vi "Device Unload.vi"(8 "error in (no error)":errorcluster, 9 "IED Name":string, 11 "SCADA in":refnum<class "SCADA.lvclass">) -> (0 "error out":errorcluster, 3 "SCADA out":refnum<class "SCADA.lvclass">)   [LabVIEW 2015, in "SCADA Core.lvlib" / "SCADA.lvclass"]
uses:
  SCADA.lvclass
  Controls/Queue Selector.ctl
  <vilib>/ActorFramework/Actor/Actor.lvclass/Actor.ctl
  SCADA.lvclass/SCADA.ctl
  <vilib>/ActorFramework/Message Enqueuer/Message Enqueuer.lvclass/Message Enqueuer.ctl
  SCADA Abstract Messages/Device Action Status Msg/Device Action Status.ctl
  <vilib>/Utility/error.llb/DialogType.ctl
  <vilib>/ActorFramework/Message Enqueuer/Enqueue.vi
  <vilib>/ActorFramework/Message Priority Queue/Priority Enqueue.vi
  <vilib>/ActorFramework/Stop Msg/Stop Msg.lvclass
  <vilib>/ActorFramework/Actor/Actor.lvclass
  SCADA Abstract Messages/Device Action Status Msg/Device Action Status Msg.lvclass
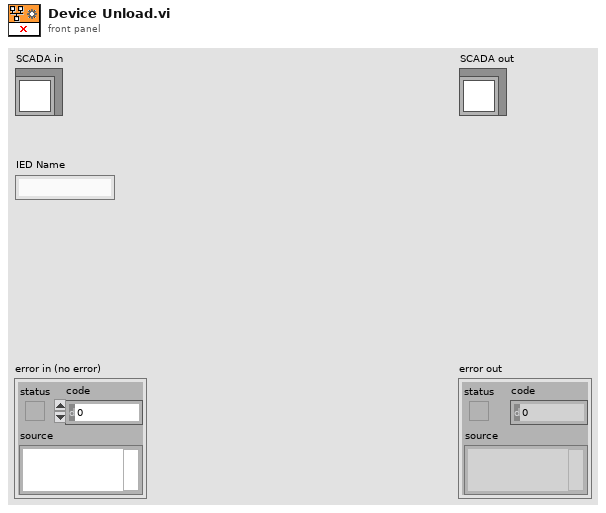
[diagram p1: front panel]
types:
  T1 = typedef "SCADA Core.lvlib/SCADA.lvclass/Queue Selector.ctl" = enum16{"IEDs", "PV", "Generators", "Wind", "Storage", "Relays"}
  T2 = typedef "SCADA Core.lvlib/Device Action Status Msg.lvclass/Device Action Status.ctl" = enum16{"Success", "Failure"}
  T3 = typedef "DialogType.ctl" = u16
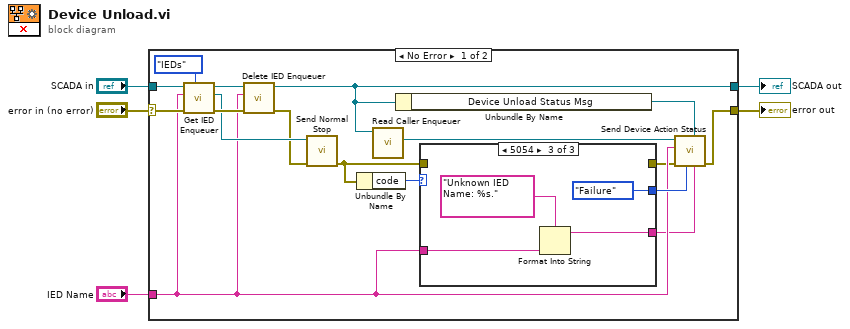
[diagram p0: block diagram]
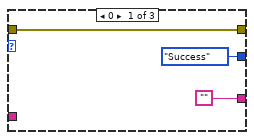
[diagram p2: hidden frame]
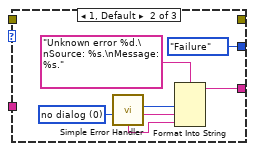
[diagram p3: hidden frame]
diagram:
  n1 = case shown="No Error" "error in (no error)" {
    selector: "error in (no error)" -> [w21 w38]
    tunnel: [w7 w38] -> w4
    tunnel: [w16 w37] -> w2
    tunnel: "SCADA in" -> [w22 w37]
    tunnel: "IED Name" -> [w10 _]
    frame No Error {
      n2 = call "Get IED Enqueuer.vi"("Queue (IEDs)"=Queue_Selector."IEDs" ("Queue"), "error in (no error)"=w21, "IED Name"=w10, "SCADA in"=w22) -> ("error out"=w19:errorcluster, "IED Enqueuer"=w18:refnum<class "Message Enqueuer.lvclass">, "SCADA out"=w20:refnum<class "SCADA.lvclass">)  [unwired: 5 in]
      n3 = call "Delete IED Enqueuer.vi"("error in (no error)"=w19, "IED Name"=w10, "SCADA in"=w20) -> ("error out"=w17:errorcluster, "SCADA out"=w16:refnum<class "SCADA.lvclass">)  [unwired: 7 in]
      n4 = call <vilib>:"Send Normal Stop.vi"("error in (no error)"=w17, "Message Enqueuer"=w18) -> ("error out"=w13:errorcluster)  [unwired: 9 in]
      n5 = Unbundle By Name(w13) -> ("code"=w12:i32)
      n6 = call <vilib>:"Read Caller Enqueuer.vi"("Actor"=w16) -> ("Caller Enqueuer"=w15:refnum<class "Message Enqueuer.lvclass">)  [unwired: 10 in]
      n7 = Unbundle By Name(w16) -> ("Device Unload Status Msg"=w14:refnum<class "Device Action Status Msg.lvclass">)
      n8 = case shown="5054" w12 {
        tunnel: w13 -> [w25 _ _]
        tunnel: [Device_Action_Status."Success" ("Status") Device_Action_Status."Failure" ("Status") Device_Action_Status."Failure" ("Status")] -> w11
        tunnel: w10 -> [_ _ w34]
        tunnel: ["" w27 w33] -> w9
        tunnel: [w25 _ _] -> w8
        frame 0 {
        }
        frame 1, Default {
          w32 = T3 0 items=["no dialog", "OK message", "continue or stop message", "OK message + warnings", "continue/stop + warnings"] ("type of dialog (OK msg:1)")
          n9 = call <vilib>:"Simple Error Handler.vi"("type of dialog (OK msg:1)"=w32) -> ("code out"=w30:i32, "source out"=w29:string, "message"=w28:string)  [unwired: 4 in, 2 out]
          n10 = Format Into String(format string="Unknown error %d.\nSource: %s.\nMessage: %s." ("Error String"), w30, w29, w28) -> (resulting string=w27:string)  [unwired: 2 in, 1 out]
        }
        frame 5054 {
          n11 = Format Into String(format string="Unknown IED Name: %s." ("Error String"), w34) -> (resulting string=w33:string)  [unwired: 2 in, 1 out]
        }
      }
      n12 = call "Send Device Action Status.vi"("error string"=w9, "Island Control Status Msg"=w14, "Status"=w11, "error in (no error)"=w8, "IED Name"=w10, "Message Enqueuer in"=w15) -> ("error out"=w7:errorcluster)  [unwired: 4 in, 1 out]
    }
    frame Error {
    }
  }
  "error out" <- w4
  "SCADA out" <- w2
